vi "Keyboard Control.vi"() -> ()   [LabVIEW 2021]
uses:
  Classes/Communication/Comm/Comm.lvclass
  <vilib>/Utility/inputDevices.llb/closeKeyboard.vi
  <vilib>/Utility/inputDevices.llb/keyboardAcquire.vi
panel:
  out "keys pressed":T1(array[ring])
  out "element":T2(ring)
  in  "Stop":bool
  out "Sensor Reading":dbl(graph)
  in  "Write":string
  out "Read":string
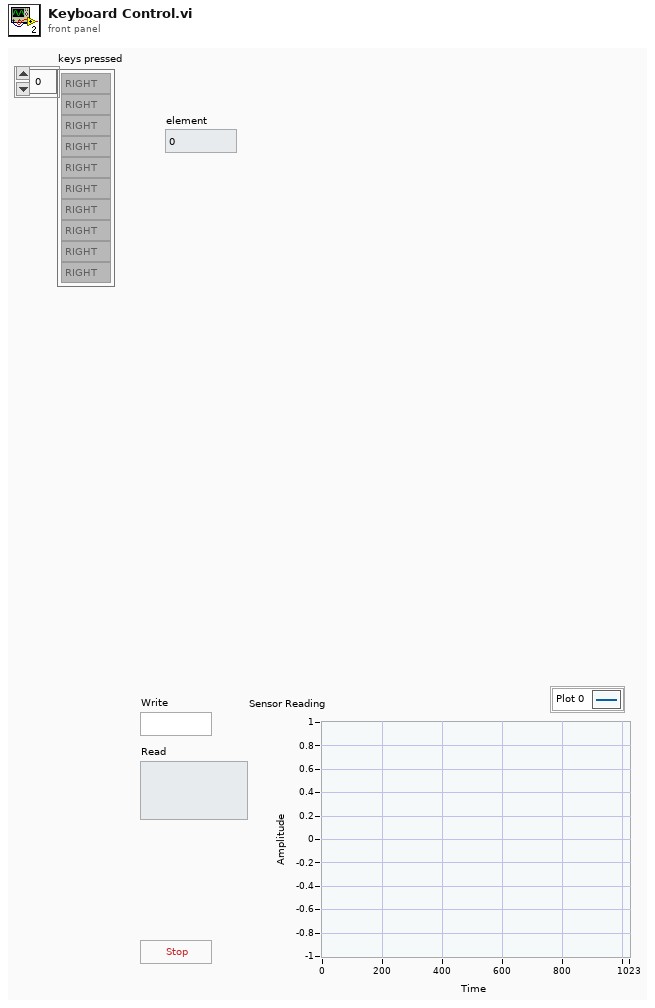
[diagram p1: front panel]
types:
  T1 = enum16{"0", "1", "2", "3", "4", "5", "6", "7", "8", "9", "A", "B", "C", "D", "E", "F", "G", "H", "I", "J", "K", "L", "M", "N", "O", "P", "Q", "R", "S", "T", "U", "V", "W", "X", "Y", "Z", "F1", "F2", "F3", "F4", "F5", "F6", "F7", "F8", "F9", "F10", "F11", "F12", "F13", "F14", "F15", "ADD", "BACK", "BACKSLASH", "CAPITAL", "COMMA", "DECIMAL", "DELETE", "DIVIDE", "DOWN", "END", "EQUALS", "ESCAPE", "GRAVE (`)", "HOME", "INSERT", "LBRACKET", "LCONTROL", "LEFT", "L ALT", "LSHIFT", "LWIN", "MINUS", "MULTIPLY", "NEXT", "NUMLOCK", "NUMPAD_0", "NUMPAD_1", "NUMPAD_2", "NUMPAD_3", "NUMPAD_4", "NUMPAD_5", "NUMPAD_6", "NUMPAD_7", "NUMPAD_8", "NUMPAD_9", "PAUSE", "PERIOD", "PRIOR (PG UP)", "RBRACKET", "RCONTROL", "RETURN", "RIGHT", "R ALT", "RSHIFT", "RWIN", "SCROLL", "SEMICOLON", "SLASH", "SPACE", "SUBTRACT", "TAB", "UP", "ENTER (num pad)", "' (quote)"}[]
  T2 = enum16{"0", "1", "2", "3", "4", "5", "6", "7", "8", "9", "A", "B", "C", "D", "E", "F", "G", "H", "I", "J", "K", "L", "M", "N", "O", "P", "Q", "R", "S", "T", "U", "V", "W", "X", "Y", "Z", "F1", "F2", "F3", "F4", "F5", "F6", "F7", "F8", "F9", "F10", "F11", "F12", "F13", "F14", "F15", "ADD", "BACK", "BACKSLASH", "CAPITAL", "COMMA", "DECIMAL", "DELETE", "DIVIDE", "DOWN", "END", "EQUALS", "ESCAPE", "GRAVE (`)", "HOME", "INSERT", "LBRACKET", "LCONTROL", "LEFT", "L ALT", "LSHIFT", "LWIN", "MINUS", "MULTIPLY", "NEXT", "NUMLOCK", "NUMPAD_0", "NUMPAD_1", "NUMPAD_2", "NUMPAD_3", "NUMPAD_4", "NUMPAD_5", "NUMPAD_6", "NUMPAD_7", "NUMPAD_8", "NUMPAD_9", "PAUSE", "PERIOD", "PRIOR (PG UP)", "RBRACKET", "RCONTROL", "RETURN", "RIGHT", "R ALT", "RSHIFT", "RWIN", "SCROLL", "SEMICOLON", "SLASH", "SPACE", "SUBTRACT", "TAB", "UP", "ENTER (num pad)", "' (quote)"}
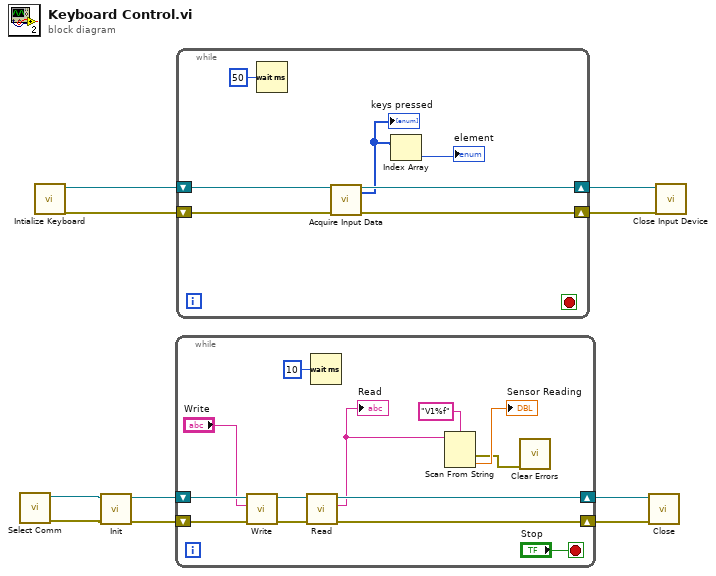
[diagram p0: block diagram]
diagram:
  n1 = call "Select Comm.vi"() -> ("error out"=w5:errorcluster, "Comm.lvclass"=w6:refnum<class "Comm.lvclass">)  [unwired: 10 in]
  n2 = call <vilib>:"Intialize Keyboard.vi"() -> ("error out"=w3:errorcluster, "device ID"=w4:refnum<k1>)  [unwired: 10 in]
  n3 = call-dynamic "Init.vi"("error in (no error)"=w5, "Comm in"=w6) -> ("error out"=w10:errorcluster, "Comm out"=w7:refnum<class "Comm.lvclass">)  [unwired: 8 in]
  n4 = while {
    shift-right: [w21] -> w8
    shift-left: w10 -> [w23]
    shift-right: [w22] -> w9
    shift-left: w7 -> [w19]
    stop <- "Stop" stop-if-true
    n5 = call-dynamic "Write.vi"("error in (no error)"=w23, "Message"="Write", "Comm in"=w19) -> ("error out"=w20:errorcluster, "Comm out"=w18:refnum<class "Comm.lvclass">)  [unwired: 7 in]
    n6 = call-dynamic "Read.vi"("error in (no error)"=w20, "Comm in"=w18) -> ("error out"=w21:errorcluster, "Message"=w15:string, "Comm out"=w22:refnum<class "Comm.lvclass">)  [unwired: 7 in]
    "Read" <- w15
    n7 = Wait (ms)(milliseconds to wait=u32 10) -> ()  [unwired: 1 out]
    n8 = Scan From String(format string="V1%f", input string=w15) -> (error out=w11:errorcluster, output 1=→"Sensor Reading":dbl)  [unwired: 3 in, 2 out]
    n9 = call <vilib>:"Clear Errors.vi"("error in (no error)"=w11) -> ()  [unwired: 5 in, 2 out]
  }
  n10 = while {
    shift-right: [w28] -> w2
    shift-left: w4 -> [w30]
    shift-right: [w27] -> w1
    shift-left: w3 -> [w29]
    stop <- _ stop-if-true
    n11 = Wait (ms)(milliseconds to wait=u32 50) -> ()  [unwired: 1 out]
    n12 = call-poly <vilib>:"Acquire Input Data.vi"("device ID"=w30, "error in (no error)"=w29) -> ("device ID"=w28:refnum<k1>, "keys pressed"=w25:T1, "error out"=w27:errorcluster)  [unwired: 15 in]
    "keys pressed" <- w25
    n13 = Index Array(array=w25) -> (element=→"element":T2)  [unwired: 1 in]
  }
  n14 = call-dynamic "Close.vi"("error in (no error)"=w8, "Comm in"=w9) -> ()  [unwired: 8 in, 2 out]
  n15 = call-poly <vilib>:"Close Input Device.vi"("error in (no error)"=w1, "device ID"=w2) -> ()  [unwired: 8 in, 1 out]
